vi "LeerPistofono.vi"(8 "error in (no error)":errorcluster, 9 "FactorCalibPistofono":dbl=1.0, 10 "clusterPistofono":T1, 11 "Pistofono in":refnum<class "Pistofono.lvclass">) -> (0 "error out":errorcluster, 2 "clusterPistofono out":T1, 3 "Pistofono out":refnum<class "Pistofono.lvclass">)   [LabVIEW 2019, in "Pistofono.lvclass"]
uses:
  Pistofono.lvclass
  Pruebas/AjustesPrevios/Controles/ClusterLecturaPistofono.ctl
  Pruebas/AjustesPrevios/AjustesPrevios.lvclass
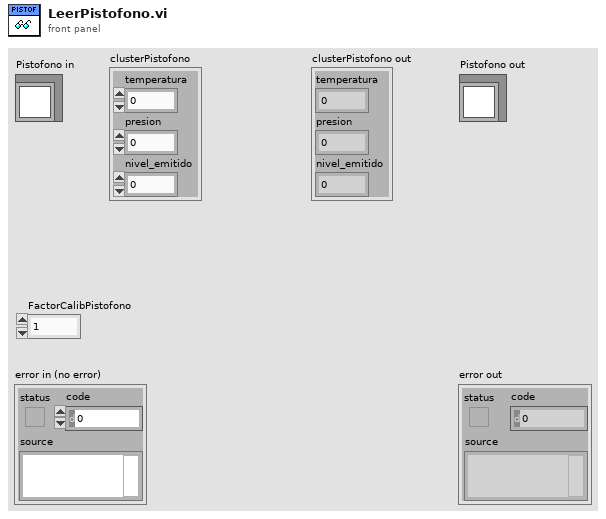
[diagram p1: front panel]
types:
  T1 = typedef "AjustesPrevios.lvclass/ClusterLecturaPistofono.ctl" = cluster{"temperatura":dbl, "presion":dbl, "nivel_emitido":dbl}
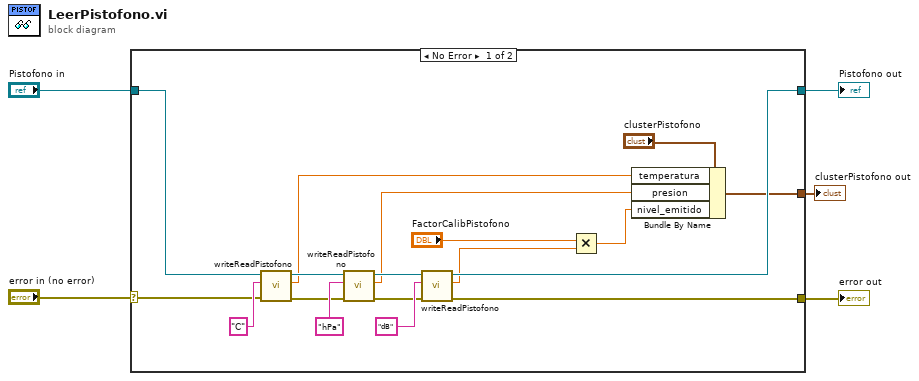
[diagram p0: block diagram]
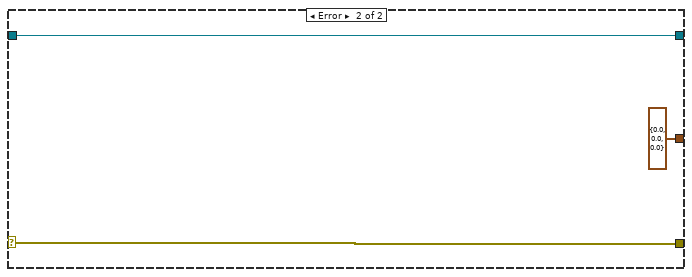
[diagram p2: hidden frame]
diagram:
  n1 = case shown="No Error" "error in (no error)" {
    selector: "error in (no error)" -> [w16 w26]
    tunnel: [w15 w26] -> w4
    tunnel: [w13 w25] -> w2
    tunnel: "Pistofono in" -> [w14 w25]
    tunnel: [w6 T1 {"temperatura"=0.0, "presion"=0.0, "nivel_emitido"=0.0} ("clusterPistofono")] -> w1
    frame No Error {
      n2 = call "writeReadPistofono.vi"("error in (no error)"=w16, "Command"="C", "Pistofono in"=w14) -> ("error out"=w18:errorcluster, "medicion (num)"=w12:dbl, "Pistofono out"=w22:refnum<class "Pistofono.lvclass">)  [unwired: 6 in]
      n3 = call "writeReadPistofono.vi"("error in (no error)"=w18, "Command"="hPa", "Pistofono in"=w22) -> ("error out"=w17:errorcluster, "medicion (num)"=w11:dbl, "Pistofono out"=w23:refnum<class "Pistofono.lvclass">)  [unwired: 6 in]
      n4 = call "writeReadPistofono.vi"("error in (no error)"=w17, "Command"="dB", "Pistofono in"=w23) -> ("error out"=w15:errorcluster, "medicion (num)"=w9:dbl, "Pistofono out"=w13:refnum<class "Pistofono.lvclass">)  [unwired: 6 in]
      n5 = Multiply(x="FactorCalibPistofono", y=w9) -> (x*y=w8:dbl)
      n6 = Bundle By Name(cluster="clusterPistofono", "temperatura"=w12, "presion"=w11, "nivel_emitido"=w8) -> (w6:T1)
    }
    frame Error {
    }
  }
  "error out" <- w4
  "Pistofono out" <- w2
  "clusterPistofono out" <- w1
